vi "Generate Error.vi"(8 "Error In":errorcluster, 10 "Arguments":string[](array[string]), 11 "DSTM Error":T1) -> (0 "Error Out":errorcluster)   [LabVIEW 2011, in "LVH-Adept.lvlib" / "DSTM.lvlib"]
uses:
  DSTM.lvlib
  Type Defs/Error.ctl
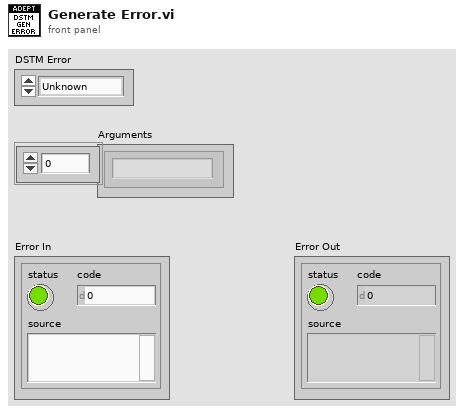
[diagram p1: front panel]
types:
  T1 = typedef "LVH-Adept.lvlib/DSTM.lvlib/Error.ctl" = enum16{"Unknown", "Enable", "Data Transfer", "Disable"}
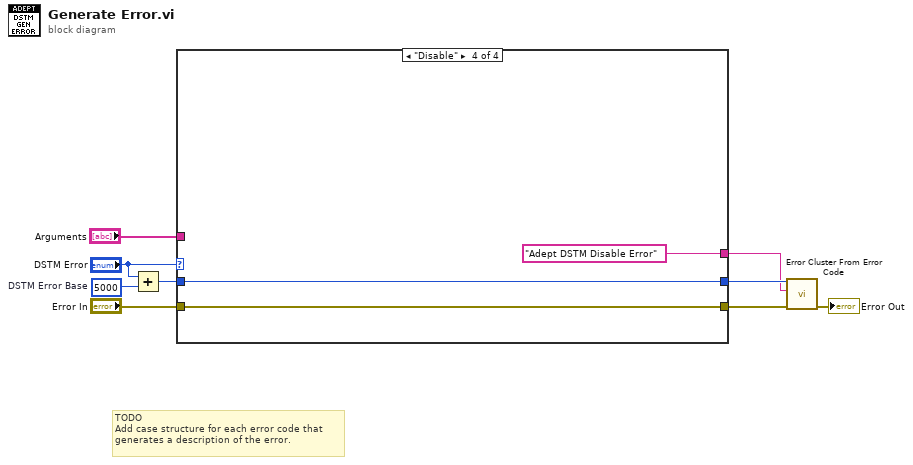
[diagram p0: block diagram]
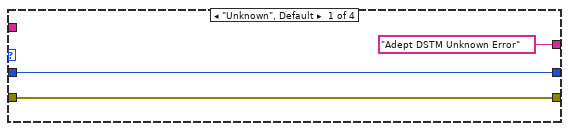
[diagram p2: hidden frame]
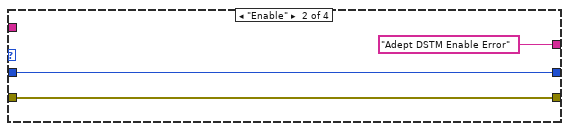
[diagram p3: hidden frame]
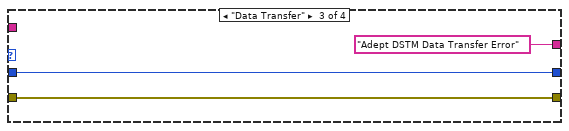
[diagram p4: hidden frame]
diagram:
  w6 = 5000  # DSTM Error Base
  # "TODO\nAdd case structure for each error code that \ngenerates a description of the error."
  n1 = Add(x="DSTM Error", y=w6) -> (x+y=w3:i32)
  n2 = case shown="\"Disable\"" "DSTM Error" {
    tunnel: [w12 w15 w18 w21] -> w8
    tunnel: "Error In" -> [w12 w15 w18 w21]
    tunnel: [w10 w13 w16 w19] -> w5
    tunnel: ["Adept DSTM Unknown Error" "Adept DSTM Enable Error" "Adept DSTM Data Transfer Error" "Adept DSTM Disable Error"] -> w4
    tunnel: w3 -> [w10 w13 w16 w19]
    tunnel: "Arguments" -> [_ _ _ _]
    frame "Unknown", Default {
    }
    frame "Enable" {
    }
    frame "Data Transfer" {
    }
    frame "Disable" {
    }
  }
  n3 = call <vilib>:"Error Cluster From Error Code.vi"("error in (no error)"=w8, "error message (\"\")"=w4, "error code (0)"=w5) -> ("error out"=→"Error Out":errorcluster)  [unwired: 6 in]
